vi "mem_test.vi"() -> ()   [LabVIEW 2010]
panel:
  out "Boolean":bool
  out "error out":errorcluster
  out "Table Control":string[][](table)
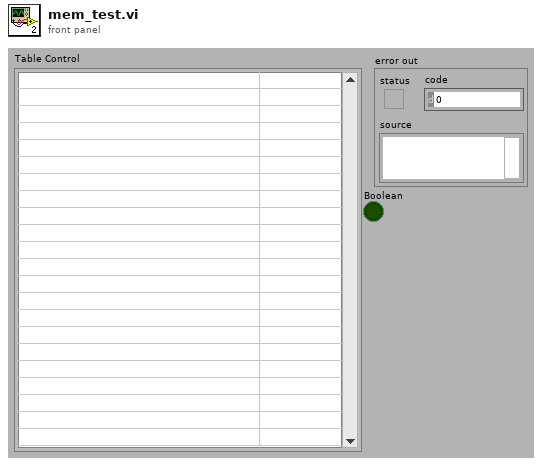
[diagram p1: front panel]
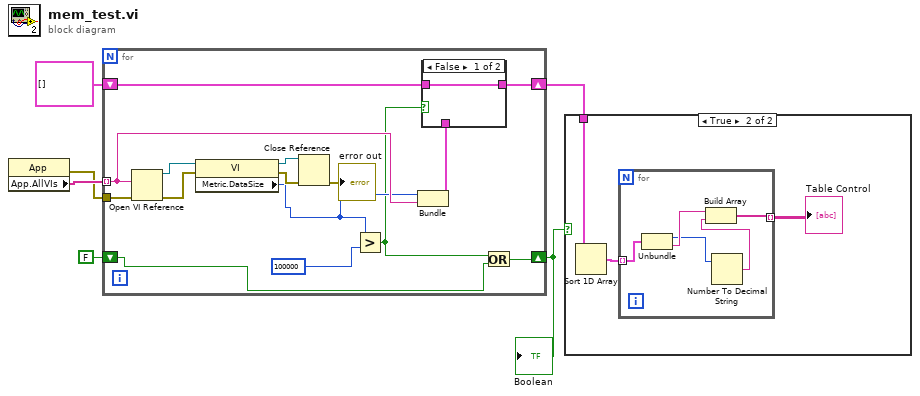
[diagram p0: block diagram]
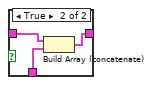
[diagram p3: hidden frame]
diagram:
  n1 = property class="App"() -> (error out=w5:errorcluster, "App.AllVIs"=w6:string[])  [unwired: 2 in, 1 out]
  n2 = for {
    tunnel: w6 -> [w16] mode=indexing
    tunnel: w5 -> [w19]
    shift-right: [w11] -> w4
    shift-left: cluster{"Metric.DataSize":u32, string}[] [] -> [w12]
    shift-right: [w9] -> w1
    shift-left: FALSE -> [w7]
    n3 = Open VI Reference(vi path=w16, error in (no error)=w19) -> (vi reference=w21:refnum<vi>, error out=w18:errorcluster)  [unwired: 4 in]
    n4 = property class="VI"(reference=w21, error in=w18) -> (reference out=w20:refnum<vi>, error out=w17:errorcluster, "Metric.DataSize"=w15:u32)
    n5 = Close Reference(reference=w20, error in (no error)=w17) -> (error out=→"error out":errorcluster)
    n6 = Greater?(x=w15, y=u32 100000) -> (0:w8:bool)
    n7 = Bundle("Metric.DataSize"=w15, w16) -> (w13:cluster{"Metric.DataSize":u32, string})  [unwired: 1 in]
    n8 = case shown="False" w8 {
      tunnel: w13 -> [_ w25]
      tunnel: w12 -> [w22 w24]
      tunnel: [w22 w23] -> w11
      frame False {
      }
      frame True {
        n9 = Build Array (concatenate)(w24, w25) -> (w23:cluster{"Metric.DataSize":u32, string}[])
      }
    }
    n10 = Or(x=w8, y=w7) -> (x .or. y?=w9:bool)
  }
  "Boolean" <- w1
  n11 = case shown="True" w1 {
    tunnel: w4 -> [_ w26]
    frame False {
    }
    frame True {
      n12 = Sort 1D Array(array=w26) -> (sorted array=w28:cluster{"Metric.DataSize":u32, string}[])
      n13 = for {
        tunnel: w28 -> [w33] mode=indexing
        tunnel: [w29] -> w27 mode=indexing
        n14 = Unbundle(w33) -> ("Metric.DataSize"=w31:u32, w32:string)
        n15 = Number To Decimal String(number=w31) -> (decimal integer string=w30:string)  [unwired: 1 in]
        n16 = Build Array(w32, w30) -> (w29:string[])
      }
      "Table Control" <- w27
    }
  }
